vi "Andor_ProcessBckgnd.vi"(8 "error in (no error)":errorcluster caption="entrée d'erreur (pas d'erreur)", 10 "Settings":T1, 11 "BackgroundIn":i32[](array[numeric])) -> (0 "error out":errorcluster caption="sortie d'erreur", 3 "BackgroundOut":i32[][](array[numeric]))   [LabVIEW 2019]
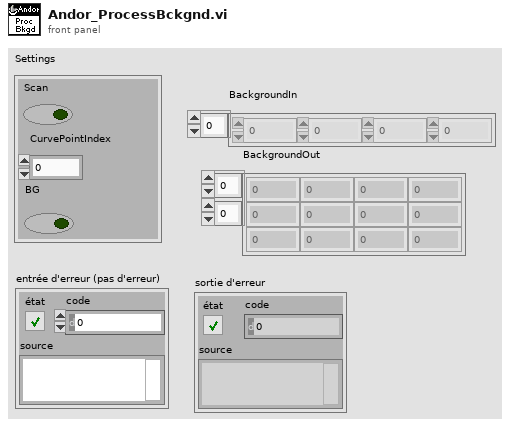
[diagram p1: front panel]
types:
  T1 = cluster{"Scan":bool, "CurvePointIndex":i32, "BG":bool}
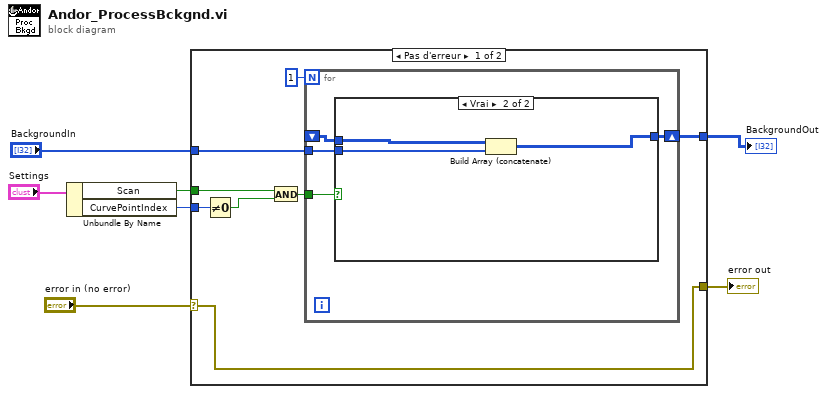
[diagram p0: block diagram]
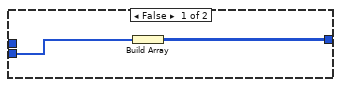
[diagram p2: hidden frame]
diagram:
  n1 = Unbundle By Name("Settings") -> ("Scan"=w3:bool, "CurvePointIndex"=w2:i32)
  n2 = case shown="Pas d'erreur" "error in (no error)" {
    selector: "error in (no error)" -> [w15 w25]
    tunnel: [w15 w25] -> w6
    tunnel: "BackgroundIn" -> [w14 _]
    tunnel: w3 -> [w8 _]
    tunnel: w2 -> [w12 _]
    tunnel: [w10 _] -> w1
    frame No Error {
      n3 = Not Equal To 0?(x=w12) -> (x != 0?=w11:bool)
      n4 = And(x=w8, y=w11) -> (x .and. y?=w13:bool)
      n5 = for {
        N: 1 -> [_]
        tunnel: w14 -> [w19]
        tunnel: w13 -> [w18]
        shift-right: [w17] -> w10
        shift-left: _ -> [w16]
        n6 = case shown="Vrai" w18 {
          tunnel: w19 -> [w20 w24]
          tunnel: [w21 w23] -> w17
          tunnel: w16 -> [_ w22]
          frame False {
            n7 = Build Array(w20) -> (w21:i32[][])
          }
          frame True {
            n8 = Build Array (concatenate)(w22, w24) -> (w23:i32[][])
          }
        }
      }
    }
    frame Error {
    }
  }
  "error out" <- w6
  "BackgroundOut" <- w1
